vi "Write Continuous Analog Waveform.vi"() -> ()   [LabVIEW 2020]
uses:
  <vilib>/DAQmx/write.llb/DAQmx Write (Analog DBL 1Chan 1Samp).vi
  <vilib>/DAQmx/create/channels.llb/DAQmx Create Channel (AI-Voltage-Basic).vi
  <vilib>/DAQmx/miscellaneous.llb/DAQmx Fill In Error Info.vi
panel:
  out "Numeric":dbl
  out "Slide":dbl(slide) scale=0.0..5.0
  in  "stop":bool
  in  "DAQmx Physical Channel":tag
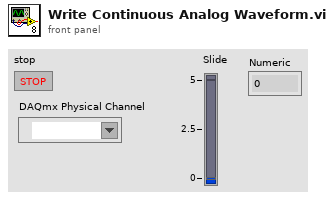
[diagram p1: front panel]
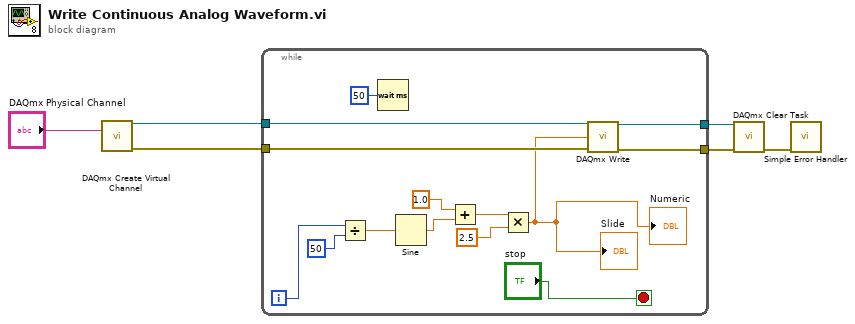
[diagram p0: block diagram]
diagram:
  n1 = call-poly <vilib>:"DAQmx Create Virtual Channel.vi"("physical channels"="DAQmx Physical Channel") -> ("task out"=w5:refnum<k21>, "error out"=w4:errorcluster)  [unwired: 13 in]
  n2 = while {
    tunnel: w5 -> [w20]
    tunnel: w4 -> [w19]
    tunnel: [w18] -> w3
    tunnel: [w17] -> w2
    i -> [w16]
    stop <- "stop" stop-if-true
    n3 = Divide(x=w16, y=50) -> (x/y=w14:dbl)
    n4 = Wait (ms)(milliseconds to wait=u32 50) -> ()  [unwired: 1 out]
    n5 = Sine(x=w14) -> (sin(x)=w13:dbl)
    n6 = Add(x=1.0, y=w13) -> (x+y=w11:dbl)
    n7 = Multiply(x=w11, y=2.5) -> (x*y=w7:dbl)
    "Slide" <- w7
    "Numeric" <- w7
    n8 = call-poly <vilib>:"DAQmx Write.vi"("task/channels in"=w20, "data"=w7, "error in"=w19) -> ("task out"=w18:refnum<k21>, "error out"=w17:errorcluster)  [unwired: 10 in, 1 out]
  }
  n9 = call <vilib>:"DAQmx Clear Task.vi"("task in"=w3, "error in"=w2) -> ("error out"=w1:errorcluster)  [unwired: 13 in]
  n10 = call <vilib>:"Simple Error Handler.vi"("error in (no error)"=w1) -> ()  [unwired: 4 in, 5 out]
